vi "CalculateThirdVoltage.vi"(8 "error out":errorcluster, 11 "voltage waveforms in":waveform(dbl)[](array[waveform])) -> (0 "error out":errorcluster, 2 "3-phases voltage waveforms":waveform(dbl)[](array[waveform]), 3 "duplicate waveforms in":waveform(dbl)[](array[waveform]))   [LabVIEW 2017, in "McsaAnalysisFunctions.lvlib"]
uses:
  <vilib>/addons/InsightCM/Utilities/Analysis/MCSA/McsaAnalysisFunctions.lvlib
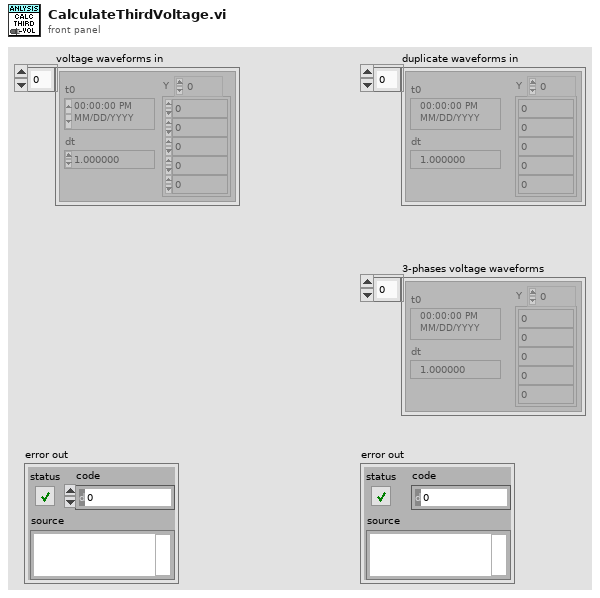
[diagram p1: front panel]
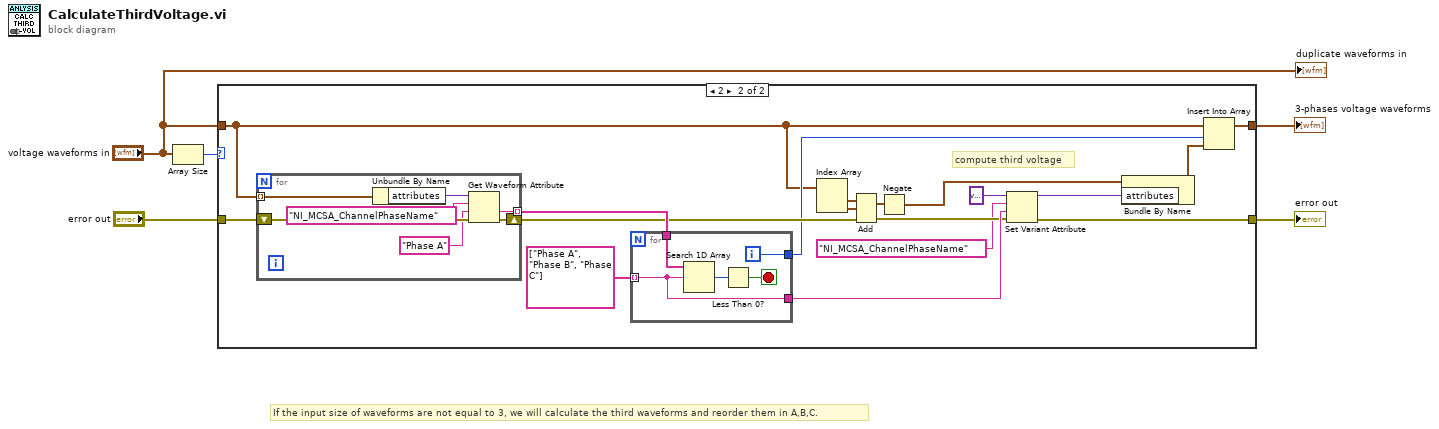
[diagram p0: block diagram]
diagram:
  # "If the input size of waveforms are not equal to 3, we will calculate the third waveforms and reorder them in A,B,C."
  n1 = Array Size(array="voltage waveforms in") -> (size(s)=w1:i32)
  n2 = case shown="2" w1 {
    tunnel: "error out" -> [w7 w24]
    tunnel: [w7 w8] -> w4
    tunnel: "voltage waveforms in" -> [w6 w10]
    tunnel: [w6 w22] -> w3
    frame 3, Default {
    }
    frame 2 {
      # "compute third voltage"
      n3 = for {
        tunnel: w10 -> [w37] mode=indexing
        tunnel: [w34] -> w25 mode=indexing
        shift-right: [w32] -> w23
        shift-left: w24 -> [w33]
        n4 = Unbundle By Name(w37) -> ("attributes"=w36:variant)
        n5 = Get Waveform Attribute(4:w33, 5:"Phase A" ("name"), 6:"NI_MCSA_ChannelPhaseName" ("name"), 7:w36) -> (0:w32:errorcluster, 1:w34:string)  [unwired: 2 out]
      }
      n6 = for {
        tunnel: w25 -> [w30]
        tunnel: string[] ["Phase A", "Phase B", "Phase C"] -> [w28] mode=indexing
        tunnel: [w28] -> w20
        tunnel: [w26] -> w11
        i -> [w26]
        stop <- w29 stop-if-true
        n7 = Search 1D Array(1D array=w30, element=w28) -> (index of element=w27:i32)  [unwired: 1 in]
        n8 = Less Than 0?(x=w27) -> (x < 0?=w29:bool)
      }
      n9 = Index Array(array=w10) -> (element #1=w13:waveform(dbl), element #2=w14:waveform(dbl))  [unwired: 2 in]
      n10 = Add(1:w14, 2:w13, 4:w23) -> (0:w15:waveform(dbl), 3:w19:errorcluster)
      n11 = Negate(x=w15) -> (-x=w16:waveform(dbl))
      n12 = Set Variant Attribute(Variant=variant ("variant"), name="NI_MCSA_ChannelPhaseName", value=w20, error in=w19) -> (Variant out=w9:variant, error out=w8:errorcluster)  [unwired: 1 out]
      n13 = Bundle By Name(cluster=w16, "attributes"=w9) -> (w12:waveform(dbl))
      n14 = Insert Into Array(array=w10, index=w11, new element=w12) -> (w22:waveform(dbl)[])
    }
  }
  "3-phases voltage waveforms" <- w3
  "error out" <- w4
  "duplicate waveforms in" <- "voltage waveforms in"
